vi "Configure Range Table (Spurious Emissions - Peak).vi"(0 "VISA resource name":refnum<visa-resource-name>, 5 "Peak Excursion":dbl[](array[numeric])=[6.0, 6.0] format="%#.6g", 7 "Peak Threshold":dbl[](array[numeric])=[-90.0, -90.0] format="%#.6g", 9 "Attenuation":dbl[](array[numeric])=[10.0, 10.0] format="%#.6g", 11 "error in (no error)":errorcluster) -> (4 "VISA resource name out":refnum<visa-resource-name>, 15 "error out":errorcluster)   [LabVIEW 2014, in "Agilent ESA PSA Series.lvlib"]
doc: "Configures the Peak and attenuation of the measurement."
uses:
  Agilent ESA PSA Series.lvlib
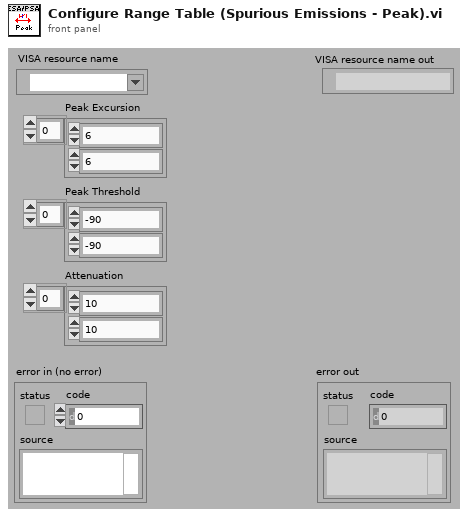
[diagram p1: front panel]
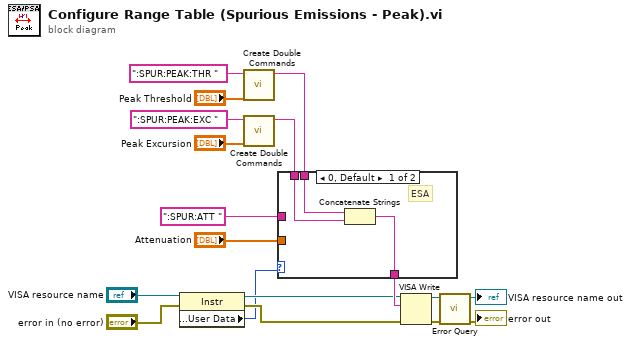
[diagram p0: block diagram]
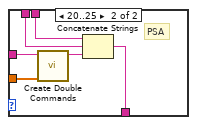
[diagram p2: hidden frame]
diagram:
  n1 = property on="Property Node" class="Instr"(reference="VISA resource name", error in="error in (no error)") -> (reference out=w3:refnum<visa-resource-name>, error out=w2:errorcluster, "General Settings:User Data"=w1:u32)
  n2 = call "Create Double Commands.vi"("Double Values"="Peak Threshold", "Commands"=":SPUR:PEAK:THR ") -> ("Result"=w7:string)  [unwired: 9 in]
  n3 = call "Create Double Commands.vi"("Double Values"="Peak Excursion", "Commands"=":SPUR:PEAK:EXC ") -> ("Result"=w6:string)  [unwired: 9 in]
  n4 = case shown="0, Default" w1 {
    tunnel: [w21 w27] -> w16
    tunnel: ":SPUR:ATT " -> [_ w26]
    tunnel: "Attenuation" -> [_ w25]
    tunnel: w7 -> [w20 w24]
    tunnel: w6 -> [w19 w23]
    frame 0, Default {
      # "ESA"
      n5 = Concatenate Strings(w20, w19) -> (w21:string)
    }
    frame 20..25 {
      # "PSA"
      n6 = call "Create Double Commands.vi"("Double Values"=w25, "Commands"=w26) -> ("Result"=w22:string)  [unwired: 9 in]
      n7 = Concatenate Strings(w24, w23, w22) -> (w27:string)
    }
  }
  n8 = VISA Write(VISA resource name=w3, write buffer=w16, error in (no error)=w2) -> (VISA resource name out=w17:refnum<visa-resource-name>, error out=w18:errorcluster)  [unwired: 1 out]
  n9 = call "Error Query.vi"("error in (no error)"=w18, "VISA resource name"=w17) -> ("error out"=→"error out":errorcluster, "VISA resource name out"=→"VISA resource name out":refnum<visa-resource-name>)  [unwired: 6 in, 2 out]
